vi "Constructor.vi"(10 "Capacity":u32) -> (3 "ErrorLog":refnum<class "LogCircularBuffer.lvclass">)   [LabVIEW 2024, in "LogCircularBuffer.lvclass"]
uses:
  LogCircularBuffer.lvclass
  LogCircularBuffer.lvclass/LogCircularBuffer.ctl
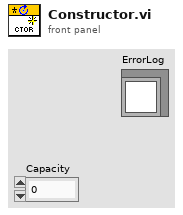
[diagram p1: front panel]
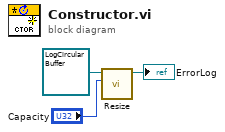
[diagram p0: block diagram]
diagram:
  n1 = call "Resize.vi"("Capacity"="Capacity", "TypedCircularBuffer in"=refnum<class "LogCircularBuffer.lvclass"> refnum ("TypedCircularBuffer.lvclass")) -> ("TypedCircularBuffer out"=→"ErrorLog":refnum<class "LogCircularBuffer.lvclass">)  [unwired: 9 in]
